vi "DataTypeNameCorrector.vi"(8 "Error In":errorcluster, 11 "Array":string[](array[string])) -> (0 "Error Out":errorcluster, 3 "Array 2":string[](array[string]))   [LabVIEW 2014]
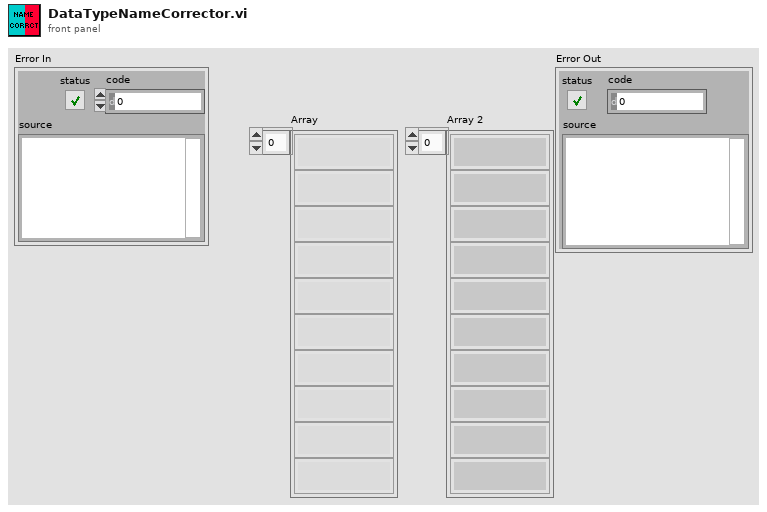
[diagram p1: front panel]
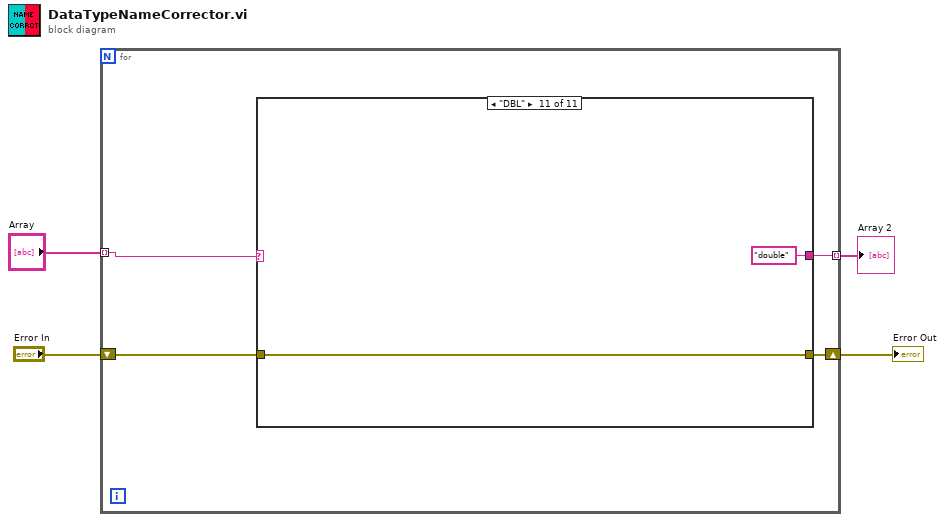
[diagram p0: block diagram]
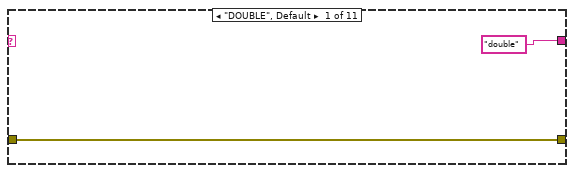
[diagram p2: hidden frame]
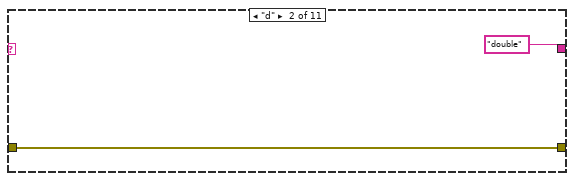
[diagram p3: hidden frame]
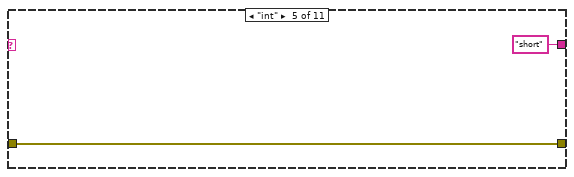
[diagram p6: hidden frame]
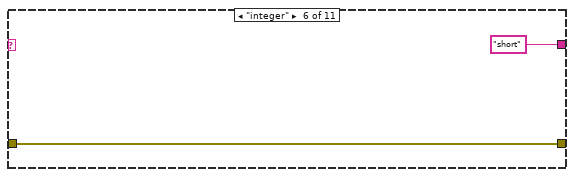
[diagram p7: hidden frame]
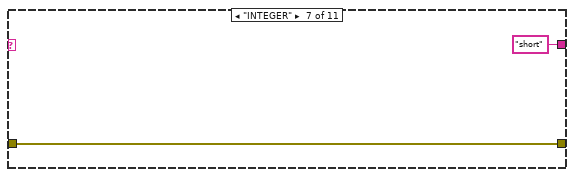
[diagram p8: hidden frame]
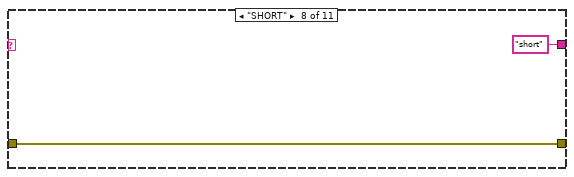
[diagram p9: hidden frame]
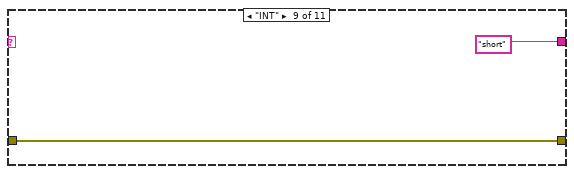
[diagram p10: hidden frame]
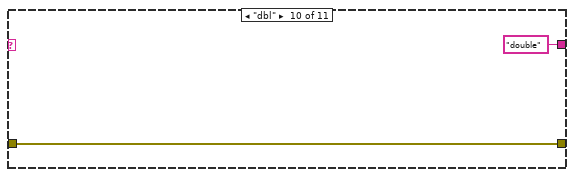
[diagram p11: hidden frame]
diagram:
  n1 = for {
    tunnel: "Array" -> [w8] mode=indexing
    tunnel: [w7] -> w3 mode=indexing
    shift-right: [w6] -> w2
    shift-left: "Error In" -> [w5]
    n2 = case shown="\"DBL\"" w8 {
      selector: w8 -> [_ _ w14 w16 _ _ _ _ _ _ _]
      tunnel: ["double" "double" w14 w16 "short" "short" "short" "short" "short" "double" "double"] -> w7
      tunnel: w5 -> [w9 w11 w13 w15 w17 w19 w21 w23 w25 w27 w29]
      tunnel: [w9 w11 w13 w15 w17 w19 w21 w23 w25 w27 w29] -> w6
      frame "DOUBLE", Default {
      }
      frame "d" {
      }
      frame "short" {
      }
      frame "double" {
      }
      frame "int" {
      }
      frame "integer" {
      }
      frame "INTEGER" {
      }
      frame "SHORT" {
      }
      frame "INT" {
      }
      frame "dbl" {
      }
      frame "DBL" {
      }
    }
  }
  "Array 2" <- w3
  "Error Out" <- w2
